vi "DrawCylinder.vi"(0 "Cylinder":T1={"Height"=0.1, "Radius"=0.1, "Color Box"=10395294, "Alpha"=1.0, "Detail"=1.0}, 1 "Name":string="Cylinder", 3 "error in (no error)":errorcluster) -> (5 "object out":refnum<vi>, 7 "error out":errorcluster)   [LabVIEW 2019]
uses:
  <vilib>/picture/3D Picture Control/Object/Create Object (name).vi
  <vilib>/picture/3D Picture Control/NI_3D Picture Control.lvlib
panel:
  out "Color":T2={"Red"=1.0, "Green"=0.0, "Blue"=0.0, "Alpha"=1.0}
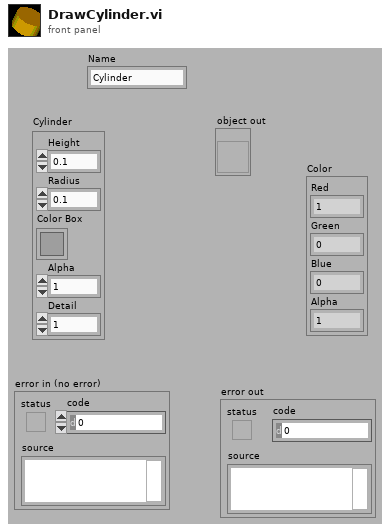
[diagram p1: front panel]
types:
  T1 = cluster{"Height":sgl, "Radius":sgl, "Color Box":u32, "Alpha":sgl, "Detail":sgl}
  T2 = cluster{"Red":sgl, "Green":sgl, "Blue":sgl, "Alpha":sgl}
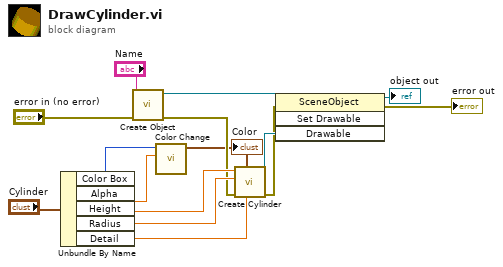
[diagram p0: block diagram]
diagram:
  n1 = Unbundle By Name("Cylinder") -> ("Color Box"=w5:u32, "Alpha"=w4:sgl, "Height"=w10:sgl, "Radius"=w9:sgl, "Detail"=w8:sgl)
  n2 = call-poly <vilib>:"Create Object.vi"("error in (no error)"="error in (no error)", "Name"="Name") -> ("error out"=w7:errorcluster, "Scene:New Object"=w13:refnum<vi>)  [unwired: 8 in]
  n3 = call <vilib>:"Color Change.vi"("Alpha"=w4, "Color"=w5) -> ("RGBA"=w3:cluster{"R":sgl, "G":sgl, "B":sgl, "A":sgl})  [unwired: 9 in]
  "Color" <- w3
  n4 = call <vilib>:"Create Cylinder.vi"("Detail"=w8, "Color"=w3, "error in (no error)"=w7, "Radius"=w9, "Height"=w10) -> ("error out"=w6:errorcluster, "New Cylinder Refnum"=w14:refnum<vi>)  [unwired: 5 in]
  n5 = invoke class="SceneObject" method="Set Drawable"(reference=w13, error in=w6, "Drawable"=w14) -> (reference out=→"object out":refnum<vi>, error out=→"error out":errorcluster)  [unwired: 1 in, 2 out]
